vi "send-multi-(SubVI).vi"(0 "read buffer":string) -> (1 "Boolean 2":bool, 2 "Numeric 4":i32, 3 "Boolean":bool, 4 "Numeric 2":i32, 5 "Numeric 3":i32, 6 "Numeric":i32, 7 "Boolean 3":bool)   [LabVIEW 2018]
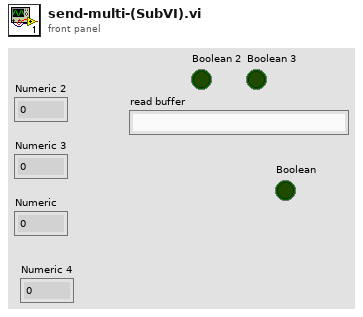
[diagram p1: front panel]
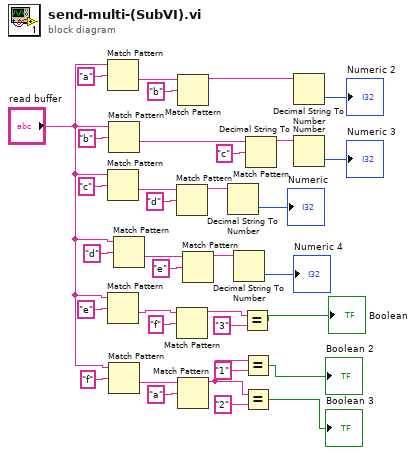
[diagram p0: block diagram]
diagram:
  n1 = Match Pattern(string="read buffer", regular expression="a") -> (after substring=w22:string)  [unwired: 1 in, 3 out]
  n2 = Match Pattern(string="read buffer", regular expression="c") -> (after substring=w28:string)  [unwired: 1 in, 3 out]
  n3 = Match Pattern(string="read buffer", regular expression="e") -> (after substring=w9:string)  [unwired: 1 in, 3 out]
  n4 = Match Pattern(string="read buffer", regular expression="b") -> (after substring=w25:string)  [unwired: 1 in, 3 out]
  n5 = Match Pattern(string="read buffer", regular expression="f") -> (after substring=w12:string)  [unwired: 1 in, 3 out]
  n6 = Match Pattern(string="read buffer", regular expression="d") -> (after substring=w19:string)  [unwired: 1 in, 3 out]
  n7 = Match Pattern(string=w28, regular expression="d") -> (before substring=w33:string)  [unwired: 1 in, 3 out]
  n8 = Match Pattern(string=w9, regular expression="f") -> (before substring=w7:string)  [unwired: 1 in, 3 out]
  n9 = Match Pattern(string=w22, regular expression="b") -> (before substring=w32:string)  [unwired: 1 in, 3 out]
  n10 = Match Pattern(string=w12, regular expression="a") -> (before substring=w5:string)  [unwired: 1 in, 3 out]
  n11 = Match Pattern(string=w19, regular expression="e") -> (before substring=w17:string)  [unwired: 1 in, 3 out]
  n12 = Decimal String To Number(string=w33) -> (number=→"Numeric":i32)  [unwired: 2 in, 1 out]
  n13 = Decimal String To Number(string=w17) -> (number=→"Numeric 4":i32)  [unwired: 2 in, 1 out]
  n14 = Equal?(x=w7, y="3") -> (x = y?=→"Boolean":bool)
  n15 = Equal?(x=w5, y="1") -> (x = y?=→"Boolean 2":bool)
  n16 = Equal?(x=w5, y="2") -> (x = y?=→"Boolean 3":bool)
  n17 = Match Pattern(string=w25, regular expression="c") -> (before substring=w30:string)  [unwired: 1 in, 3 out]
  n18 = Decimal String To Number(string=w32) -> (number=→"Numeric 2":i32)  [unwired: 2 in, 1 out]
  n19 = Decimal String To Number(string=w30) -> (number=→"Numeric 3":i32)  [unwired: 2 in, 1 out]
